vi "SW_Update_radial_segmentation_variable_info.vi"(3 "error in (no error)":errorcluster, 4 "NewVal":T19 caption="New radial segmentation" {"BORDER"."N segments BORDER" min=1 max=12; "MIDFIELD"."N segments MIDFIELD" max=8; "CENTER"."Radius, mm CENTER" min=5 step=1}, 5 "Settings cluster (local) in":T1 {"Calibration parameters"."True frame time, s" format="%.10g"; "Calibration parameters"."Disp. calibration info"."Speed, µl per ms" format="%.3g"; "Calibration parameters"."True FPS" format="%.10g"; "Calibration parameters"."Timing calibration sw/hw" format="%.10g"; "Conditions presets array"."Specifier(s)"."Validity criteria(s)"."Validity value" min=0.0 step=0.1 format="%.2g"; "Conditions presets array"."Specifier(s)"."Value" step=1.0 format="%#.2g"; "Recording and saving"."Data post-processing"."Order" min=3 max=11 step=2; "Recording and saving"."Data post-processing"."Length" min=5 max=301 step=2; "Geometry"."Cage type" items=["Round", "Square", "Donut-maze", "T-maze", "Sociability maze", ""]}) -> (0 "error out":errorcluster, 2 "Settings cluster (local) out":T1 {"Calibration parameters"."True frame time, s" format="%.10g"; "Calibration parameters"."Disp. calibration info"."Speed, µl per ms" format="%.3g"; "Calibration parameters"."True FPS" format="%.10g"; "Calibration parameters"."Timing calibration sw/hw" format="%.10g"; "Conditions presets array"."Specifier(s)"."Validity criteria(s)"."Validity value" min=0.0 step=0.1 format="%.2g"; "Conditions presets array"."Specifier(s)"."Value" step=1.0 format="%#.2g"; "Recording and saving"."Data post-processing"."Order" min=3 max=11 step=2; "Recording and saving"."Data post-processing"."Length" min=5 max=301 step=2; "Geometry"."Cage type" items=["Round", "Square", "Donut-maze", "T-maze", "Sociability maze", ""]})   [LabVIEW 2018, in "Tracker.lvlib"]
uses:
  Tracker.lvlib
  Controls/CTL_Cage_radial_segmentation.ctl
  Controls/CTL_Settings_cluster.ctl
  Controls/CTL_Histogram_parameters.ctl
  Controls/CTL_Filter_selector.ctl
  Controls/CTL_Acquisition_speed_selector.ctl
  Controls/CTL_Segmented_plot_parameters_2.ctl
  Libraries/Cage Diagram/Typedefs/CTL_Cage_type.ctl
  Controls/CTL_Cage_all_segmentation_params_set.ctl
  Controls/CTL_IO_params_cluster.ctl
  Controls/CTL_Conditions_Array.ctl
  Controls/CTL_Conditions_Cluster.ctl
  Controls/CTL_Condition_type.ctl
  Controls/CTL_Comparison_type.ctl
  Controls/CTL_Validity_check_criteria.ctl
  Controls/CTL_Response_info.ctl
  Controls/CTL_Condition_response_type.ctl
  Controls/CTL_Reponse_port_info.ctl
  Controls/CTL_Calibration_parameters.ctl
  Controls/CTL_Dispenser_calibration_info.ctl
  Controls/CTL_Segmented_plot_parameters_2_(round_d1).ctl
  Common_Resources.lvlib
  Libraries/Cage Diagram/Cage Diagram.lvlib
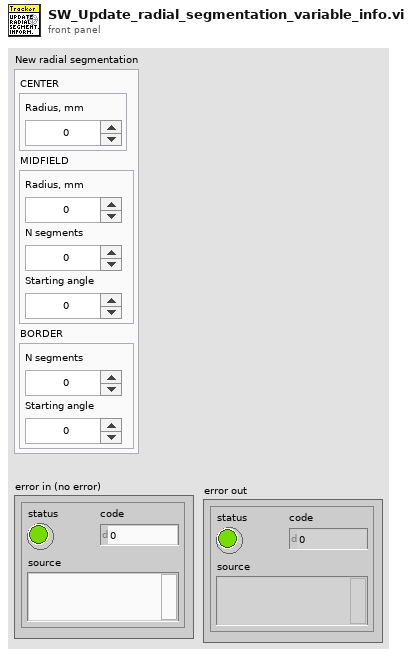
[diagram p1: front panel]
types:
  T1 = typedef "Common_Resources.lvlib/CTL_Settings_cluster.ctl" = cluster{"Defaults":cluster{"Default User":dbl, "VISA Resource Name ":string, "Histogram parameters":T2}, "Recording and saving":cluster{"Researcher name":string, "Name prefix":string, "Data post-processing":T3, "Stop at":dbl, "\"Stop at\" enabled":bool, "Default save folder path":path, "Acquisition FPS":T4}, "Geometry":T5, "IO parameters":T8, "Conditions presets array":T9, "Calibration parameters":T17, "Settings loaded OK":bool}
  T2 = typedef "Common_Resources.lvlib/CTL_Histogram_parameters.ctl" = cluster{"max":dbl, "min":dbl, "# bins":i32, "threshold":dbl, "thr. type":enum16{"higher accepted", "lower accepted"}}
  T3 = typedef "Common_Resources.lvlib/CTL_Filter_selector.ctl" = cluster{"Filter type":enum16{"None", "Savitzky-Golay"}, "Length":i32, "Order":i32}
  T4 = typedef "Common_Resources.lvlib/CTL_Acquisition_speed_selector.ctl" = enum16{"Max", "Optimal", "Eco"}
  T5 = typedef "Common_Resources.lvlib/CTL_Segmented_plot_parameters_2.ctl" = cluster{"Sensor board size":enum16{"", "Large"}, "Bridge swap":bool, "Twisted neck":bool, "Bridge H. offset":sgl, "Bridge V. offset":sgl, "Magnets orientation":sgl, "Cage type":T6, "Cage parameters":T7}
  T6 = typedef "Cage Diagram.lvlib/CTL_Cage_type.ctl" = u16
  T7 = typedef "Common_Resources.lvlib/CTL_Cage_all_segmentation_params_set.ctl" = cluster{"Round":variant, "Square":variant, "Donut-maze":variant, "T-maze":variant, "Sociability-maze":variant}
  T8 = typedef "Common_Resources.lvlib/CTL_IO_params_cluster.ctl" = cluster{"IO general config.":u16, "IO 1 configuration":u16, "IO 2 configuration":u16, "IO 3 configuration":u16, "IO 4 configuration":u16, "Activate ext. RS-232":u16, "IO inversion config.":u16, "Sync capability":u8}
  T9 = typedef "Common_Resources.lvlib/CTL_Conditions_Array.ctl" = T10[]
  T10 = typedef "Common_Resources.lvlib/CTL_Conditions_Cluster.ctl" = cluster{"Enabled":bool, "Name":string, "Specifier(s)":cluster{"Specifier enabled":bool, "Condition type":T11, "Comparison type":T12, "Value":dbl, "Validity criteria(s)":cluster{"V. check enabled":bool, "Criteria":T13, "Validity value":dbl}[]}[], "Response":T14, "Has been set":bool}
  T11 = typedef "Common_Resources.lvlib/CTL_Condition_type.ctl" = enum16{"Speed", "Zone", "Angle to wall"}
  T12 = typedef "Common_Resources.lvlib/CTL_Comparison_type.ctl" = enum16{"Less", "Less or Equal", "Equal", "Greater or Equal", "Greater", "Not Equal"}
  T13 = typedef "Common_Resources.lvlib/CTL_Validity_check_criteria.ctl" = enum16{"Running bout (seconds)", "Running bout (meters)"}
  T14 = typedef "Common_Resources.lvlib/CTL_Response_info.ctl" = cluster{"Response type":T15, "TTL port":T16, "TTL pulse length, ms":dbl}
  T15 = typedef "Common_Resources.lvlib/CTL_Condition_response_type.ctl" = enum16{"None", "Air puff", "Liquid reward", "TTL pulse", "TTL pulse (ubr)", "TTL signal"}
  T16 = typedef "Common_Resources.lvlib/CTL_Reponse_port_info.ctl" = enum16{"Port 1", "Port 2", "Port 3", "Port 4"}
  T17 = typedef "Common_Resources.lvlib/CTL_Calibration_parameters.ctl" = cluster{"Timing calibration sw/hw":dbl, "True FPS":dbl, "True frame time, s":dbl, "Disp. calibration info":T18}
  T18 = typedef "Common_Resources.lvlib/CTL_Dispenser_calibration_info.ctl" = cluster{"Channel":u8, "Speed, µl per ms":dbl}[]
  T19 = typedef "Common_Resources.lvlib/CTL_Cage_radial_segmentation.ctl" = cluster{"CENTER":cluster{"Radius, mm CENTER":u16}, "MIDFIELD":cluster{"Radius, mm MIDFIELD":u16, "N segments MIDFIELD":u8, "Starting angle MIDFIELD":i16}, "BORDER":cluster{"N segments BORDER":u8, "Starting angle BORDER":i16}}
  T20 = typedef "Common_Resources.lvlib/CTL_Segmented_plot_parameters_2_(round_d1).ctl" = cluster{"Cage diameter, mm":u16, "Starting angle BORDER":i16, "Starting angle MIDFIELD":i16, "Radius, mm MIDFIELD":u16, "Radius, mm CENTER":u16, "N segments BORDER":u8, "N segments MIDFIELD":u8, "R-gap, mm":sgl}
  T21 = cluster{"Radius, mm MIDFIELD":u16, "N segments MIDFIELD":u8, "Starting angle MIDFIELD":i16}
  T22 = cluster{"N segments BORDER":u8, "Starting angle BORDER":i16}
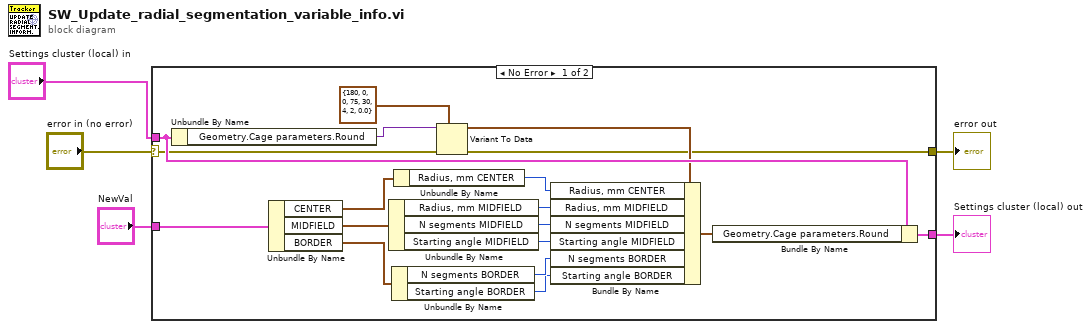
[diagram p0: block diagram]
diagram:
  n1 = case shown="No Error" "error in (no error)" {
    selector: "error in (no error)" -> [w6 w25]
    tunnel: "NewVal" -> [w23 _]
    tunnel: [w22 w24] -> w4
    tunnel: "Settings cluster (local) in" -> [w20 w24]
    tunnel: [w7 w25] -> w2
    frame No Error {
      n2 = Unbundle By Name(w20) -> ("Geometry.Cage parameters.Round"=w17:variant)
      n3 = Unbundle By Name(w23) -> ("CENTER"=w16:cluster{"Radius, mm CENTER":u16}, "MIDFIELD"=w15:T21, "BORDER"=w14:T22)
      n4 = Unbundle By Name(w15) -> ("Radius, mm MIDFIELD"=w12:u16, "N segments MIDFIELD"=w11:u8, "Starting angle MIDFIELD"=w10:i16)
      n5 = Unbundle By Name(w14) -> ("N segments BORDER"=w9:u8, "Starting angle BORDER"=w8:i16)
      n6 = Unbundle By Name(w16) -> ("Radius, mm CENTER"=w13:u16)
      n7 = Variant To Data(error in=w6, type=T20 {"Cage diameter, mm"=180, "Starting angle BORDER"=0, "Starting angle MIDFIELD"=0, "Radius, mm MIDFIELD"=75, "Radius, mm CENTER"=30, "N segments BORDER"=4, "N segments MIDFIELD"=2, "R-gap, mm"=0.0} ("Radial segmentation parameters"), Variant=w17) -> (data=w19:T20, error out=w7:errorcluster)
      n8 = Bundle By Name(cluster=w19, "Radius, mm CENTER"=w13, "Radius, mm MIDFIELD"=w12, "N segments MIDFIELD"=w11, "Starting angle MIDFIELD"=w10, "N segments BORDER"=w9, "Starting angle BORDER"=w8) -> (w21:T20)
      n9 = Bundle By Name(cluster=w20, "Geometry.Cage parameters.Round"=w21) -> (w22:T1)
    }
    frame Error {
    }
  }
  "Settings cluster (local) out" <- w4
  "error out" <- w2
